vi "CoerceData.vi"(6 "Old DO sizes":i32, 7 "Old AO sizes":i32, 8 "error in (no error)":errorcluster, 9 "New DO sizes":i32, 10 "New AO sizes":i32, 11 "NI Card in":refnum<class "NI Card.lvclass">) -> (0 "error out":errorcluster, 3 "NI Card out":refnum<class "NI Card.lvclass">)   [LabVIEW 2013, in "NI Card.lvclass"]
doc: "If the number of AOs or DOs is changed, this function coerces the NI card device data to match. Added chanels will be initialized with \"0\"s. If channel number decreases, data columns will be removed from the end of DOs/AOs as appropriate. (It's a big pain to do something smarter!)"
uses:
  NI Card.lvclass
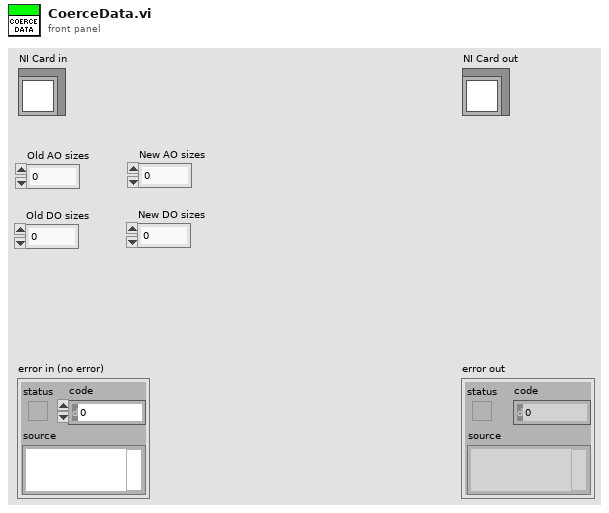
[diagram p1: front panel]
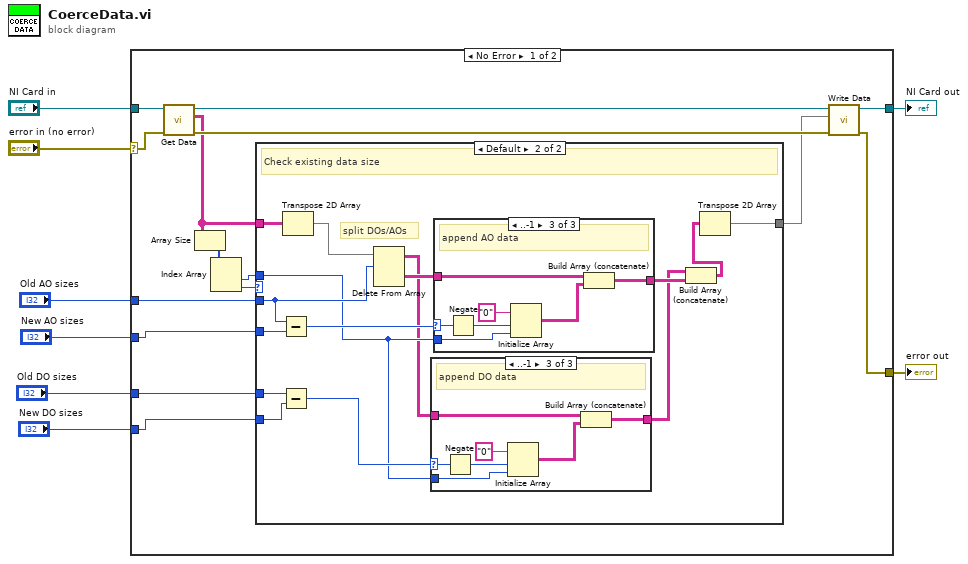
[diagram p0: block diagram]
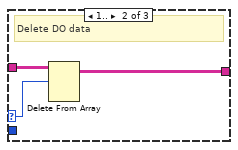
[diagram p4: hidden frame]
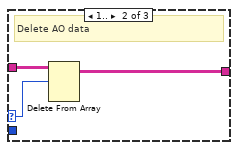
[diagram p6: hidden frame]
diagram:
  n1 = case shown="No Error" "error in (no error)" {
    selector: "error in (no error)" -> [w18 w63]
    tunnel: [w19 w63] -> w7
    tunnel: [w20 w62] -> w5
    tunnel: "NI Card in" -> [w21 w62]
    tunnel: "Old AO sizes" -> [w14 _]
    tunnel: "New AO sizes" -> [w13 _]
    tunnel: "Old DO sizes" -> [w12 _]
    tunnel: "New DO sizes" -> [w11 _]
    frame No Error {
      n2 = call-dynamic "Get Data.vi"("error in (no error)"=w18, "Device in"=w21) -> ("error out"=w22:errorcluster, "Table Indicator"=w16:string[][], "Device out"=w23:refnum<class "NI Card.lvclass">)  [unwired: 6 in]
      n3 = Array Size(array=w16) -> (size(s)=w17:i32[])
      n4 = Index Array(array=w17) -> (element #1=w9:i32, element #2=w10:i32)  [unwired: 2 in]
      n5 = case shown="Default" w10 {
        tunnel: [w24 w38] -> w15
        tunnel: w16 -> [w24 w33]
        tunnel: w14 -> [_ w34]
        tunnel: w13 -> [_ w39]
        tunnel: w12 -> [_ w32]
        tunnel: w11 -> [_ w35]
        tunnel: w9 -> [_ w31]
        frame 0 {
          # "Default Data will be called within Add Device next."
          # "New device added; leave data empty"
        }
        frame Default {
          # "split DOs/AOs"
          # "Check existing data size"
          n6 = Subtract(x=w34, y=w39) -> (x-y=w37:i32)
          n7 = Subtract(x=w32, y=w35) -> (x-y=w36:i32)
          n8 = Transpose 2D Array(2D array=w33) -> (transposed array=w30:string[][])
          n9 = Delete From Array(array=w30, length=w34) -> (deleted portion=w29:string[][], array with subset deleted=w28:string[][])  [unwired: 2 in]
          n10 = case shown="..-1" w36 {
            selector: w36 -> [_ w42 w50]
            tunnel: w28 -> [w40 w43 w46]
            tunnel: [w40 w41 w44] -> w26
            tunnel: w31 -> [_ _ w48]
            frame 0, Default {
              # "No DO changes"
            }
            frame 1.. {
              # "Delete DO data"
              n11 = Delete From Array(array=w43, length=w42) -> (array with subset deleted=w41:string[][])  [unwired: 2 in, 1 out]
            }
            frame ..-1 {
              # "append DO data"
              n12 = Negate(x=w50) -> (-x=w49:i32)
              n13 = Initialize Array("0", w49, w48) -> (w45:string[][])
              n14 = Build Array (concatenate)(w46, w45) -> (w44:string[][])
            }
          }
          n15 = case shown="..-1" w37 {
            selector: w37 -> [_ w53 w61]
            tunnel: w29 -> [w51 w54 w57]
            tunnel: [w51 w52 w55] -> w27
            tunnel: w31 -> [_ _ w59]
            frame 0, Default {
              # "No AO changes"
            }
            frame 1.. {
              # "Delete AO data"
              n16 = Delete From Array(array=w54, length=w53) -> (array with subset deleted=w52:string[][])  [unwired: 2 in, 1 out]
            }
            frame ..-1 {
              # "append AO data"
              n17 = Negate(x=w61) -> (-x=w60:i32)
              n18 = Initialize Array("0", w60, w59) -> (w56:string[][])
              n19 = Build Array (concatenate)(w57, w56) -> (w55:string[][])
            }
          }
          n20 = Build Array (concatenate)(w26, w27) -> (w25:string[][])
          n21 = Transpose 2D Array(2D array=w25) -> (transposed array=w38:string[][])
        }
      }
      n22 = call-dynamic "Write Data.vi"("error in (no error)"=w22, "Data"=w15, "Device in"=w23) -> ("error out"=w19:errorcluster, "Device Out"=w20:refnum<class "NI Card.lvclass">)  [unwired: 7 in]
    }
    frame Error {
    }
  }
  "error out" <- w7
  "NI Card out" <- w5
